vi "SPI Engine Top.vi"(8 "error in":errorcluster, 10 "SPI Read Data":T3, 11 "SPI API References":T2={"DLU To SPI Engine Data FIFO"="DLU To SPI Engine Data", "SPI Engine to DLU Data FIFO"="SPI Engine to DLU Data", "Data to SPI Engine (Cache) Register"="Data to SPI Engine (Cache)", "SPI PHY Settings to SPI Engine (Cahche) Register"="SPI PHY Settings to SPI Engine (Cache)"}) -> (0 "error out":errorcluster, 1 "Chip Select ID":u8, 2 "SPI DIO Output":T4, 3 "SPI API References Out":T2={"DLU To SPI Engine Data FIFO"="DLU To SPI Engine Data", "SPI Engine to DLU Data FIFO"="SPI Engine to DLU Data", "Data to SPI Engine (Cache) Register"="Data to SPI Engine (Cache)", "SPI PHY Settings to SPI Engine (Cahche) Register"="SPI PHY Settings to SPI Engine (Cache)"})   [LabVIEW 2014]
uses:
  user.lib/_NI SPI IP/FPGA/Controllers/Public/Spi Master Outputs.ctl
  user.lib/_NI SPI IP/FPGA/Controllers/Public/Spi Master Inputs.ctl
  Controls/Internal Data (SPI API).ctl
  Controls/SPI Response Information.ctl
  user.lib/_NI SPI IP/FPGA/Controllers/NI SPI IP (FPGA).lvlib
panel:
  out "Output Data":T1
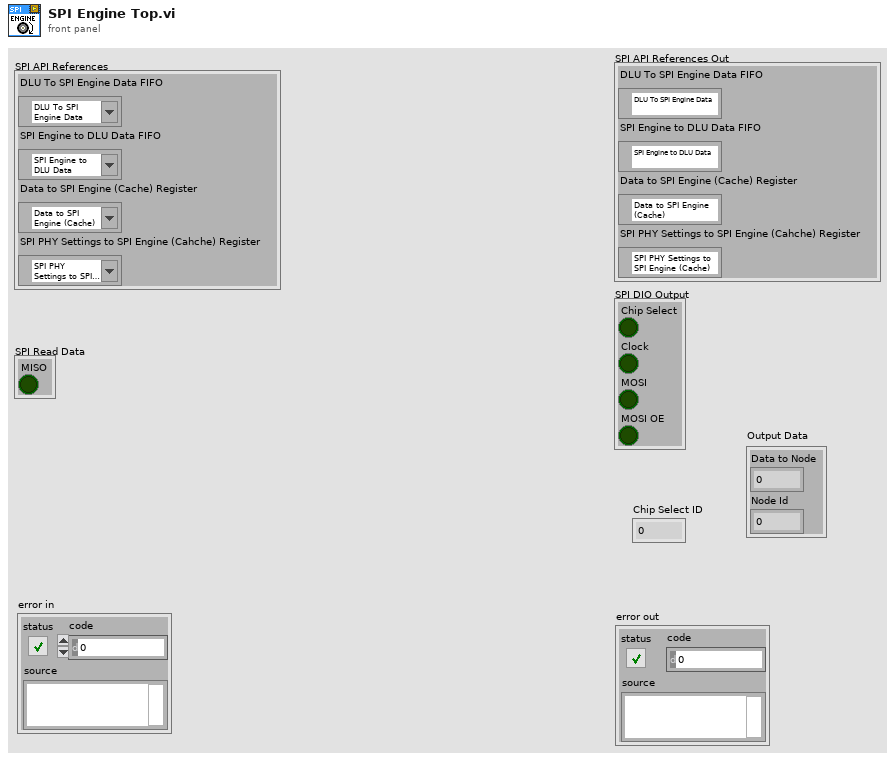
[diagram p1: front panel]
types:
  T1 = typedef "SPI Response Information.ctl" = cluster{"Data to Node":u64, "Node Id":u16}
  T2 = typedef "Internal Data (SPI API).ctl" = cluster{"DLU To SPI Engine Data FIFO":refnum<k21>, "SPI Engine to DLU Data FIFO":refnum<k21>, "Data to SPI Engine (Cache) Register":refnum<k21>, "SPI PHY Settings to SPI Engine (Cahche) Register":refnum<k21>}
  T3 = typedef "NI SPI IP (FPGA).lvlib/Spi Master Inputs.ctl" = cluster{"MISO":bool}
  T4 = typedef "NI SPI IP (FPGA).lvlib/Spi Master Outputs.ctl" = cluster{"Chip Select":bool, "Clock":bool, "MOSI":bool, "MOSI OE":bool}
  T5 = typedef "SPI Transaction Packet.ctl" = cluster{"Chip Select ID":u8, "SPI Data":u64, "Start Strobe":bool, "SPI PHY Settings":cluster{"Divide Value":u8, "Transfer Length (bits)":u8, "CS Asserted Polarity":bool, "Clock Polarity (CPOL)":bool, "Clock Phase (CPHA)":bool, "Lengthen MISO Setup":bool, "Direction Change Bit":u8, "MOSI Starts as Output":bool, "Tristatable MOSI":bool}}
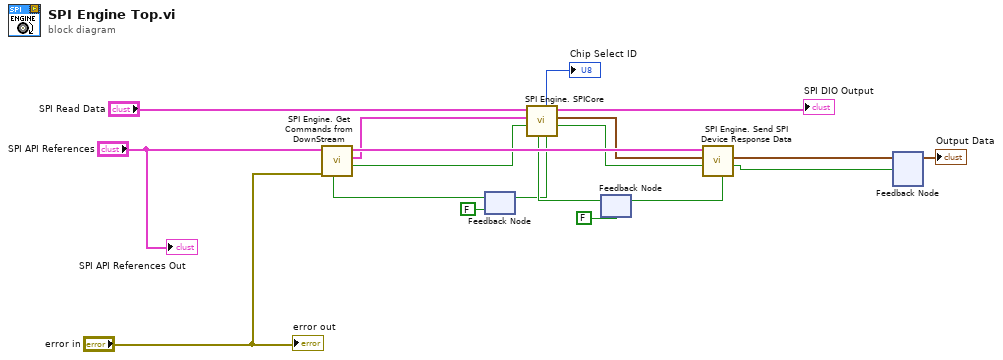
[diagram p0: block diagram]
diagram:
  n1 = feedback #1(FALSE ("ready for input")) -> (w17:bool)
  n2 = call "SPI Engine. Get Commands from DownStream.vi"("Ready for Output"=w17, "error in"="error in", "Private Data In"="SPI API References") -> ("Output Valid"=w4:bool, "SPI Transaction Packet"=w5:T5, "Private Data Out"=w15:T2)  [unwired: 4 in, 2 out]
  n3 = feedback #2(FALSE ("Ready for Input")) -> (w12:bool)
  n4 = call "SPI Engine. SPICore.vi"("Ready for Output"=w12, "Input Valid"=w4, "SPI Information In"=w5, "SPI DIO Input"="SPI Read Data") -> ("Output Valid"=w2:bool, "SPI Output Data"=w8:T1, "SPI DIO Output"=→"SPI DIO Output":T4, "Ready For Input"=w9:bool, "Chip Select ID"=→"Chip Select ID":u8)  [unwired: 3 in]
  n5 = feedback-in #1(w9) -> ()
  n6 = call "SPI Engine. Send SPI Device Response Data.vi"("Input Valid"=w2, "Input Data"=w8, "Private Data In"=w15) -> ("New Data Sent?"=w3:bool, "Output Data"=w6:T1, "Ready for Input"=w11:bool)  [unwired: 5 in, 1 out]
  n7 = feedback-in #2(w11) -> ()
  n8 = feedback-in #3(w6, w3) -> ()
  n9 = feedback #3() -> (→"Output Data":T1)  [unwired: 1 in]
  "error out" <- "error in"
  "SPI API References Out" <- "SPI API References"
